vi "Iteration Metric - X Correlation.vi"(0 "reference in":refnum<class "AdvSigProc.lvclass">, 5 "error in (no error)":errorcluster, 6 "Weighting":u16(ring) items=["biased (N)", "unbiased (N-k)"], 7 "Reference Signal":i32, 9 "Response Signal":i32) -> (14 "reference out":refnum<class "AdvSigProc.lvclass">, 19 "error out":errorcluster)   [LabVIEW 2020, in "AdvSigProc.lvclass"]
uses:
  AdvSigProc.lvclass
  protected/Iteration Metrics.ctl
  API/GSwFormDSP_class/GSwFormDSP.lvclass
  <vilib>/addons/_Advanced Signal Processing/NI_AdvSigProcTSA.lvlib
  <vilib>/addons/Time Series Analysis/Correlation and Spectral Analysis.llb/TSA Cross-Correlation Function (Waveform).vi
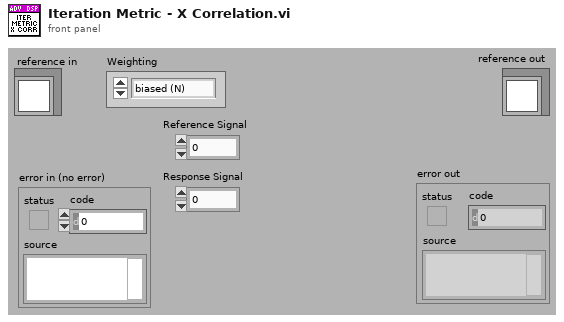
[diagram p1: front panel]
types:
  T1 = typedef "AdvSigProc.lvclass/Iteration Metrics.ctl" = cluster{"Name":string, "Max":dbl, "Min":dbl, "Values History":dbl[]}
  T2 = typedef "AdvSigProc.lvclass/ObjectAttributesRef.ctl" = refnum<data-value>
  T3 = typedef "AdvSigProc.lvclass/ObjectAttributes.ctl" = cluster{"Time Data":cluster{"New Time Data Obj?":bool, "GSwFormDSP":refnum<class "GSwFormDSP.lvclass">}, "LMS Parameters":T4}
  T4 = typedef "AdvSigProc.lvclass/LMS.ctl" = cluster{"adaptive filter Ref":refnum<k20>, "Filtered Signals":refnum<class "GSwFormDSP.lvclass">, "Filter Coefs":dbl[], "Input Parameters":T5, "Iteration Metrics":T1[]}
  T5 = typedef "AdvSigProc.lvclass/LMS Input Parameters.ctl" = cluster{"Type":enum16{"Normalized LMS", "LMS", "FIR Sign LMS", "FIR Fast Block LMS", "RLS", "QR - RLS"}, "Filter Class":enum16{"Noise Cancelling (BGN Ref)", "Noise Cancelling (Speech Ref)"}, "Filter Length":i32, "µ Parameters":cluster{"Type":enum16{"User Input", "Auto µ"}, "step size":dbl}, "Iterations":cluster{"Current":i32, "Maximum":i32}}
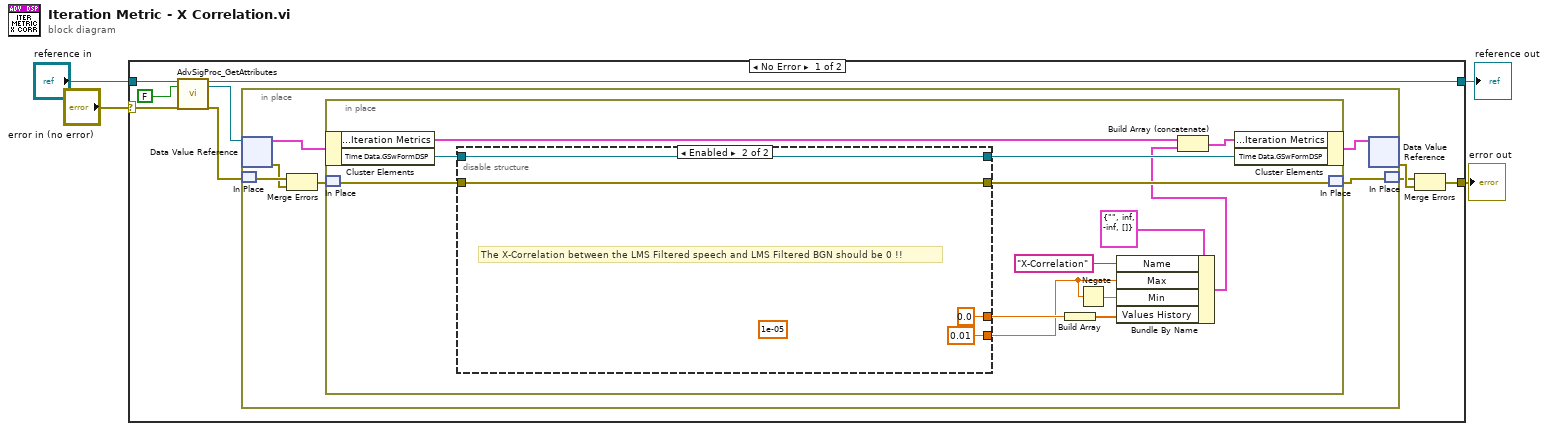
[diagram p0: block diagram]
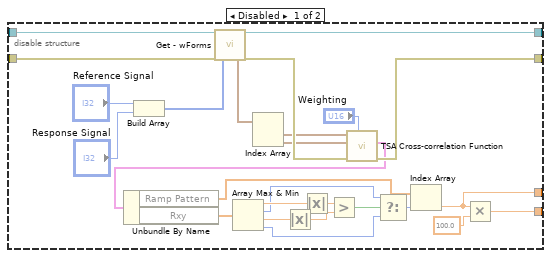
[diagram p2: hidden frame]
diagram:
  n1 = case shown="No Error" "error in (no error)" {
    selector: "error in (no error)" -> [w9 w64]
    tunnel: [w13 w64] -> w3
    tunnel: [w8 w63] -> w1
    tunnel: "reference in" -> [w11 w63]
    frame No Error {
      n2 = call "AdvSigProc_GetAttributes.vi"("reference in"=w11, "return data? (T)"=FALSE, "error in (no error)"=w9) -> ("reference out"=w8:refnum<class "AdvSigProc.lvclass">, "attributes ref"=w7:T2, "error out"=w6:errorcluster)  [unwired: 13 in, 1 out]
      n3 = in-place {
        n4 = in-place-dvr #1(w7) -> (w18:T3, w16:errorcluster)
        n5 = in-place-match #2(w6) -> (w17:errorcluster)
        n6 = Merge Errors(w17, w16) -> (w15:errorcluster)
        n7 = in-place {
          n8 = in-place-cluster #3(w18) -> ("LMS Parameters.Iteration Metrics"=w32:T1[], "Time Data.GSwFormDSP"=w28:refnum<class "GSwFormDSP.lvclass">)
          n9 = in-place-match #4(w15) -> (w26:errorcluster)
          n10 = disable-structure shown="Enabled" {
            disable-tunnel: w28 -> [w56 w60]
            disable-tunnel: [w55 w60] -> w27
            disable-tunnel: w26 -> [w54 w59]
            disable-tunnel: [w37 w59] -> w25
            disable-tunnel: [w35 0.0] -> w24
            disable-tunnel: [w34 0.01] -> w21
            frame Disabled {
              n11 = Build Array("Reference Signal", "Response Signal") -> (w53:i32[])
              n12 = call-dynamic "Get - wForms.vi"("reference in"=w56, "error in (no error)"=w54, "Indexes (Empty = ALL)"=w53) -> ("wForms"=w40:waveform(dbl)[], "reference out"=w55:refnum<class "GSwFormDSP.lvclass">, "error out"=w41:errorcluster)  [unwired: 13 in, 1 out]
              n13 = Index Array(array=w40) -> (element #1=w39:waveform(dbl), element #2=w38:waveform(dbl))  [unwired: 2 in]
              n14 = call-poly <vilib>:"TSA Cross-correlation Function.vi"("weighting"="Weighting", "error in (no error)"=w41, "Yt"=w38, "Xt"=w39) -> ("error out"=w37:errorcluster, "correlogram"=w33:cluster{"Ramp Pattern":dbl[], "Rxy":dbl[]})  [unwired: 1 in, 5 out]
              n15 = Unbundle By Name(w33) -> ("Ramp Pattern"=w49:dbl[], "Rxy"=w43:dbl[])
              n16 = Array Max & Min(array=w43) -> (max value=w51:dbl, max index (indices)=w46:i32, min value=w52:dbl, min index (indices)=w47:i32)
              n17 = Absolute Value(x=w52) -> (abs(x)=w45:dbl)
              n18 = Absolute Value(x=w51) -> (abs(x)=w44:dbl)
              n19 = Greater?(x=w44, y=w45) -> (0:w50:bool)
              n20 = Select(t=w46, s=w50, f=w47) -> (s? t:f=w48:i32)
              n21 = Index Array(array=w49, index=w48) -> (element=w35:dbl)
              n22 = Multiply(x=w35, y=100.0) -> (x*y=w34:dbl)
            }
            frame Enabled {
              (unwired) 1e-05
              # "The X-Correlation between the LMS Filtered speech and LMS Filtered BGN should be 0 !!"
            }
          }
          n23 = Build Array(w24) -> (w23:dbl[])
          n24 = Negate(x=w21) -> (-x=w20:dbl)
          n25 = Bundle By Name(cluster=T1 {"Name"="", "Max"=inf, "Min"=-inf, "Values History"=[]} ("Iteration Metric"), "Name"="X-Correlation", "Max"=w21, "Min"=w20, "Values History"=w23) -> (w22:T1)
          n26 = Build Array (concatenate)(w32, w22) -> (w31:T1[])
          n27 = in-place-cluster #3("LMS Parameters.Iteration Metrics"=w31, "Time Data.GSwFormDSP"=w27) -> (w19:T3)
          n28 = in-place-match #4(w25) -> (w14:errorcluster)
        }
        n29 = in-place-dvr #1(w19) -> (w12:errorcluster)  [unwired: 1 out]
        n30 = in-place-match #2(w14) -> (w5:errorcluster)
      }
      n31 = Merge Errors(w5, w12) -> (w13:errorcluster)
    }
    frame Error {
    }
  }
  "error out" <- w3
  "reference out" <- w1
